vi "ICM Parsers Path.vi"() -> (0 "error out":errorcluster, 3 "ICM Parsers Path":path)   [LabVIEW 2015]
doc: "ICM Parsers Path.vi\n\nThis VI defines where the ICM Parsers directory is located.\n\nInstrument Communication Module Version 1.0\nSeptember, 2017 Original Code Consulting David Thomson\n www.originalcode.com"
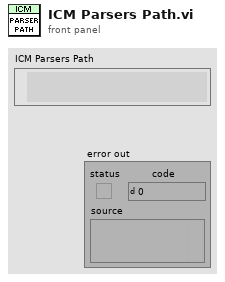
[diagram p1: front panel]
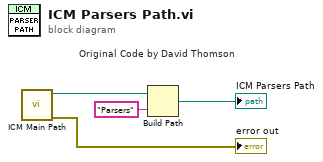
[diagram p0: block diagram]
diagram:
  w3 = "Parsers"  # Original Code by David Thomson
  n1 = call "ICM Main Path.vi"() -> ("error out"=→"error out":errorcluster, "ICM Path"=w2:path)  [unwired: 10 in]
  n2 = Build Path(base path=w2, name or relative path=w3) -> (appended path=→"ICM Parsers Path":path)
